vi "artificialHorizon.vi"(9 "pitch":dbl, 10 "yaw":dbl, 11 "roll":dbl) -> (2 "horizon picture":picture)   [LabVIEW 2014]
panel:
  in  "acceleration":dbl
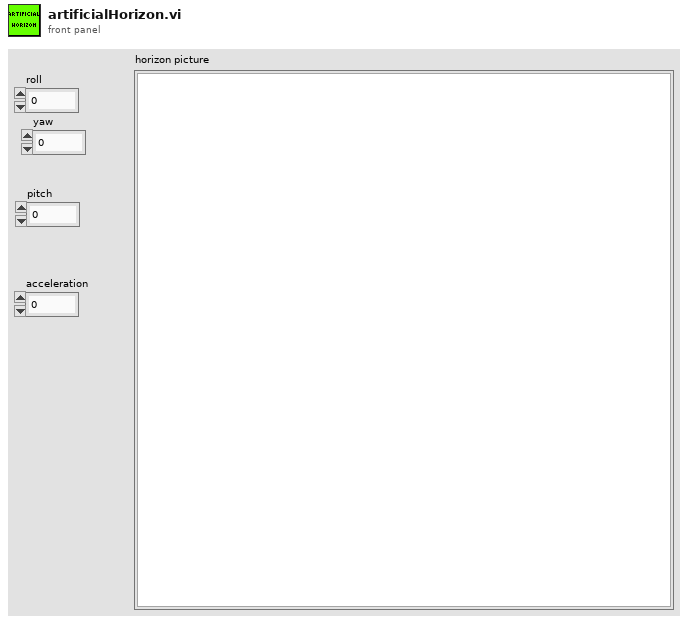
[diagram p1: front panel]
types:
  T1 = cluster{"horizontal":bool, "left/top":bool, "draw bar":bool, "line color":u32, "text color(black)":u32}
  T2 = cluster{"left":i16, "top":i16, "right":i16, "bottom":i16}
  T3 = cluster{"coordinate 1":i16, "value 1":dbl, "coordinate 2":i16, "value 2":dbl, "log?(F)":bool, "fmt and prec":cluster{"format":enum8{"Decimal", "Scientific", "Engineering", "Binary", "Octal", "Hex"}, "precision":u8}}
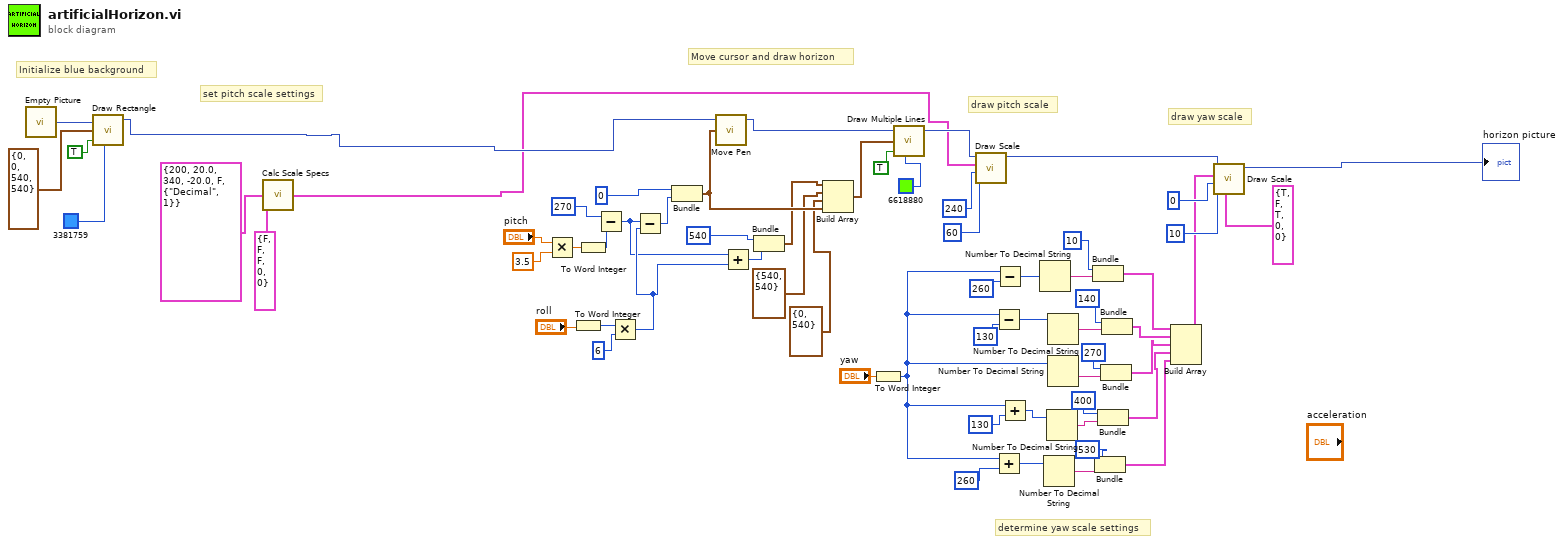
[diagram p0: block diagram]
diagram:
  # "determine yaw scale settings"
  # "draw yaw scale"
  # "set pitch scale settings"
  # "draw pitch scale"
  # "Move cursor and draw horizon"
  # "Initialize blue background"
  n1 = call "Empty Picture"() -> ("empty picture"=w62:picture)
  n2 = call <vilib>:"Draw Rectangle.vi"("picture"=w62, "rect"=T2 {"left"=0, "top"=0, "right"=540, "bottom"=540}, "fill?(F)"=TRUE, "color(black)"=u32 3381759) -> ("new picture"=w2:picture)  [unwired: 5 in]
  n3 = call <vilib>:"Calc Scale Specs.vi"("scale definition"=T3 {"coordinate 1"=200, "value 1"=20.0, "coordinate 2"=340, "value 2"=-20.0, "log?(F)"=FALSE, "fmt and prec"={"format"=enum."Decimal", "precision"=1}}, "scale attributes"=T1 {"horizontal"=FALSE, "left/top"=FALSE, "draw bar"=FALSE, "line color"=0, "text color(black)"=0}) -> ("scale specs"=w1:cluster{"coordinate":i16, "label":string}[])  [unwired: 7 in]
  n4 = Multiply(x="pitch", y=3.5) -> (x*y=w3:dbl)
  n5 = To Word Integer(number="roll") -> (16bit integer=w56:i16)
  n6 = To Word Integer(number=w3) -> (16bit integer=w38:i16)
  n7 = Subtract(x=i16 270, y=w38) -> (x-y=w45:i16)
  n8 = Multiply(x=w56, y=i16 6) -> (x*y=w58:i16)
  n9 = Subtract(x=w45, y=w58) -> (x-y=w42:i16)
  n10 = Bundle(i16 0, w42) -> (w51:cluster{i16, i16})  [unwired: 1 in]
  n11 = call <vilib>:"Move Pen.vi"("new position"=w51, "picture"=w2) -> ("new picture"=w44:picture)  [unwired: 3 in]
  n12 = Add(x=w45, y=w58) -> (x+y=w46:i16)
  n13 = Bundle(i16 540, w46) -> (w48:cluster{i16, i16})  [unwired: 1 in]
  n14 = Build Array(w48, cluster{i16, i16} {540, 540}, cluster{i16, i16} {0, 540}, w51) -> (w52:cluster{i16, i16}[])
  n15 = To Word Integer(number="yaw") -> (16bit integer=w22:i16)
  n16 = call <vilib>:"Draw Multiple Lines.vi"("picture"=w44, "line endpoints"=w52, "fill?(F)"=TRUE, "color(black)"=u32 6618880) -> ("new picture"=w53:picture)  [unwired: 5 in]
  n17 = call <vilib>:"Draw Scale.vi"("tick length(3)"=i16 60, "constant coordinate"=i16 240, "scale specs"=w1, "picture"=w53) -> ("new picture"=w33:picture)  [unwired: 7 in]
  n18 = Subtract(x=w22, y=i16 130) -> (x-y=w21:i16)
  n19 = Add(x=w22, y=i16 260) -> (x+y=w28:i16)
  n20 = Subtract(x=w22, y=i16 260) -> (x-y=w29:i16)
  n21 = Add(x=w22, y=i16 130) -> (x+y=w26:i16)
  n22 = Number To Decimal String(number=w29) -> (decimal integer string=w20:string)  [unwired: 1 in]
  n23 = Number To Decimal String(number=w28) -> (decimal integer string=w17:string)  [unwired: 1 in]
  n24 = Number To Decimal String(number=w26) -> (decimal integer string=w18:string)  [unwired: 1 in]
  n25 = Number To Decimal String(number=w21) -> (decimal integer string=w19:string)  [unwired: 1 in]
  n26 = Number To Decimal String(number=w22) -> (decimal integer string=w30:string)  [unwired: 1 in]
  n27 = Bundle(i16 10, w20) -> (w11:cluster{i16, string})  [unwired: 1 in]
  n28 = Bundle(i16 530, w17) -> (w7:cluster{i16, string})  [unwired: 1 in]
  n29 = Bundle(i16 400, w18) -> (w8:cluster{i16, string})  [unwired: 1 in]
  n30 = Bundle(i16 270, w30) -> (w9:cluster{i16, string})  [unwired: 1 in]
  n31 = Bundle(i16 140, w19) -> (w10:cluster{i16, string})  [unwired: 1 in]
  n32 = Build Array(w11, w10, w9, w8, w7) -> (w6:cluster{i16, string}[])
  n33 = call <vilib>:"Draw Scale.vi"("scale attributes"=T1 {"horizontal"=TRUE, "left/top"=FALSE, "draw bar"=TRUE, "line color"=0, "text color(black)"=0}, "tick length(3)"=i16 10, "constant coordinate"=i16 0, "scale specs"=w6, "picture"=w33) -> ("new picture"=→"horizon picture":picture)  [unwired: 6 in]
